vi "Test Case Runner.vi"(0 "Problem":T1, 1 "Numeric 2":dbl, 2 "Numeric Array 2":dbl[](array[numeric]), 3 "String 2":string, 4 "String Array 2":string[](array[string]), 5 "Iterator":i32, 8 "TestCases Folder":path, 9 "Send Input?":bool) -> (15 "Numeric":dbl, 16 "Numeric Array":dbl[](array[numeric]), 17 "String":string, 18 "String Array":string[](array[string]), 19 "Accepted":bool)   [LabVIEW 2014]
uses:
  Main Contest/Problem.ctl
  <vilib>/Utility/file.llb/Read From Spreadsheet File (string).vi
  <vilib>/Utility/file.llb/Read From Spreadsheet File (DBL).vi
panel:
  out "E":path=path "C:/Users/Justin/Desktop/LabVIEW-Rank/Offline Judge/TestCases/Test A.csv"
  out "D":path=path "C:/Users/Justin/Desktop/LabVIEW-Rank/Offline Judge/TestCases/Test A.csv"
  out "C":path=path "C:/Users/Justin/Desktop/LabVIEW-Rank/Offline Judge/TestCases/Test A.csv"
  out "B":path=path "C:/Users/Justin/Desktop/LabVIEW-Rank/Offline Judge/TestCases/Test A.csv"
  out "A":path=path "C:/Users/Justin/Desktop/LabVIEW-Rank/Offline Judge/TestCases/Test A.csv"
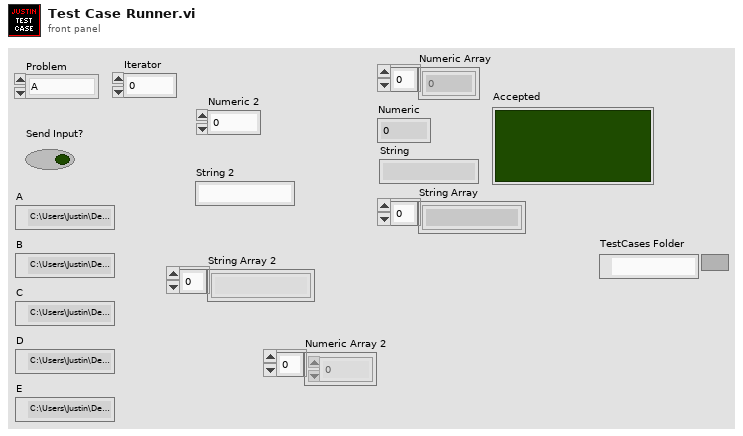
[diagram p1: front panel]
types:
  T1 = typedef "Problem.ctl" = enum16{"A", "B", "C", "D", "E"}
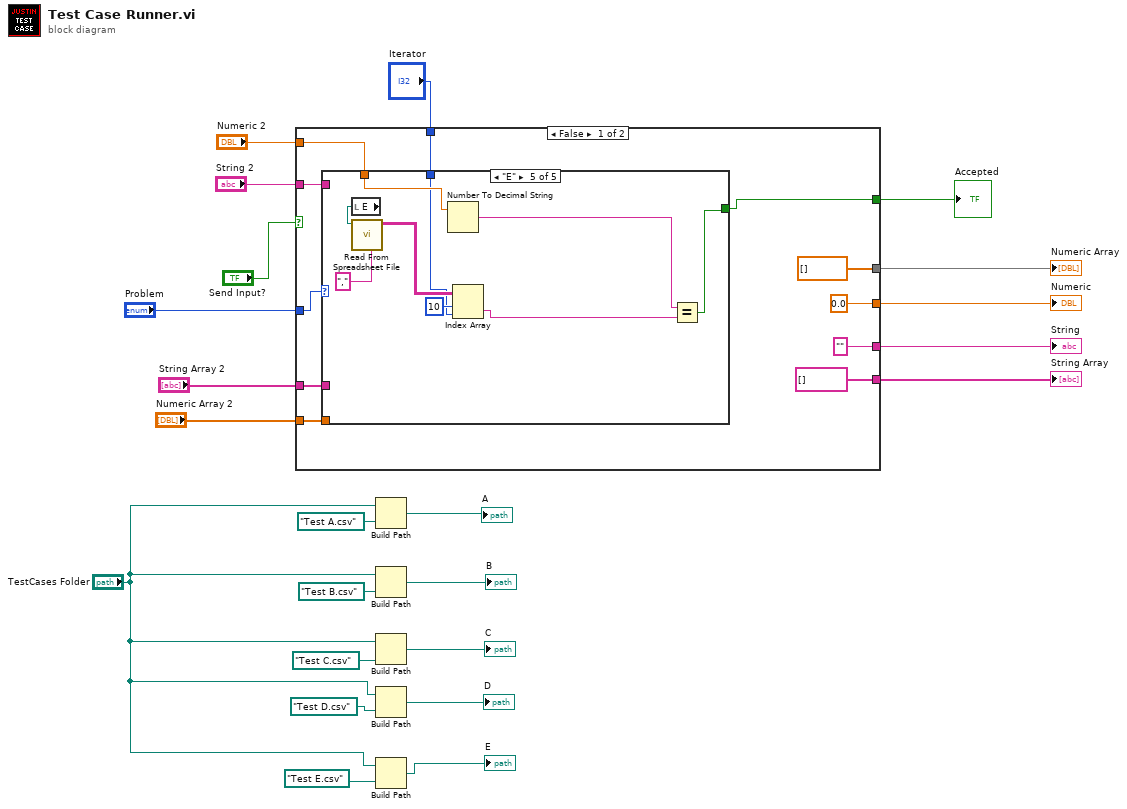
[diagram p0: block diagram]
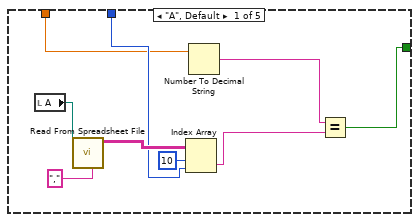
[diagram p2: hidden frame]
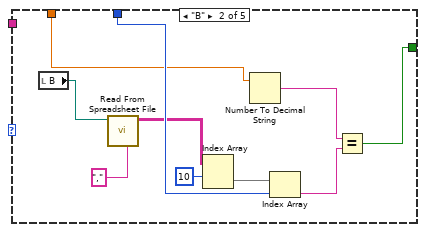
[diagram p3: hidden frame]
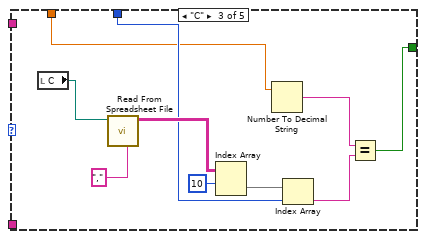
[diagram p4: hidden frame]
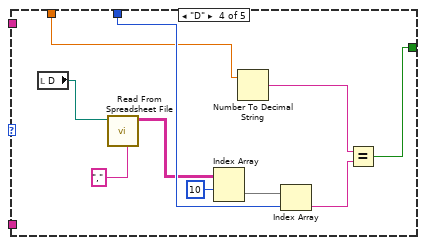
[diagram p5: hidden frame]
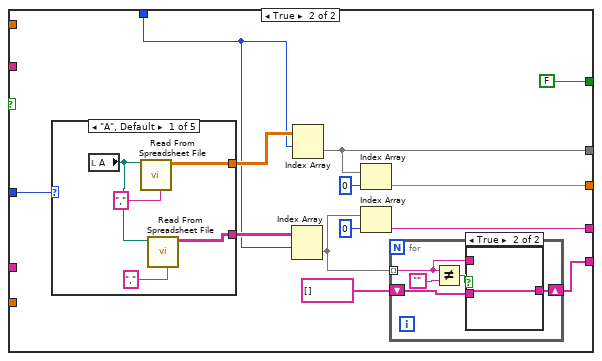
[diagram p6: hidden frame]
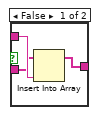
[diagram p7: hidden frame]
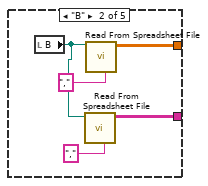
[diagram p8: hidden frame]
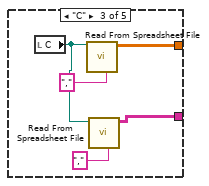
[diagram p9: hidden frame]
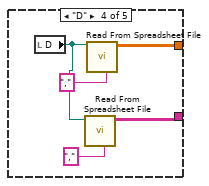
[diagram p10: hidden frame]
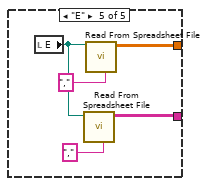
[diagram p11: hidden frame]
diagram:
  n1 = case shown="False" "Send Input?" {
    tunnel: "Problem" -> [w34 w95]
    tunnel: [w24 FALSE] -> w21
    tunnel: "Iterator" -> [w25 w88]
    tunnel: [dbl[] [] ("all rows") w92] -> w19
    tunnel: [0.0 w90] -> w18
    tunnel: [string[] [] ("all rows") w83] -> w16
    tunnel: ["" ("String") w86] -> w17
    tunnel: "Numeric 2" -> [w29 _]
    tunnel: "String Array 2" -> [w28 _]
    tunnel: "Numeric Array 2" -> [w27 _]
    tunnel: "String 2" -> [w26 _]
    frame False {
      n2 = case shown="\"E\"" w34 {
        tunnel: w29 -> [w36 w46 w56 w64 w79]
        tunnel: w28 -> [_ _ _ _ _]
        tunnel: w27 -> [_ _ _ _ _]
        tunnel: w26 -> [_ _ _ _ _]
        tunnel: w25 -> [w39 w49 w58 w69 w75]
        tunnel: [w40 w47 w57 w67 w81] -> w24
        frame "A", Default {
          n3 = local read "A"() -> (w43:path)
          n4 = call-poly <vilib>:"Read From Spreadsheet File.vi"("delimiter (\\t)"="," ("delimiter (\\t)"), "file path (dialog if empty)"=w43) -> ("all rows"=w42:string[][])  [unwired: 5 in, 4 out]
          n5 = Index Array(array=w42, index (row)=10, index (col)=w39) -> (element=w38:string)
          n6 = Number To Decimal String(number=w36) -> (decimal integer string=w35:string)  [unwired: 1 in]
          n7 = Equal?(x=w35, y=w38) -> (x = y?=w40:bool)
        }
        frame "B" {
          n8 = local read "B"() -> (w53:path)
          n9 = call-poly <vilib>:"Read From Spreadsheet File.vi"("delimiter (\\t)"="," ("delimiter (\\t)"), "file path (dialog if empty)"=w53) -> ("all rows"=w48:string[][])  [unwired: 5 in, 4 out]
          n10 = Index Array(array=w48, index (row)=10) -> (element=w51:string[])  [unwired: 1 in]
          n11 = Number To Decimal String(number=w46) -> (decimal integer string=w45:string)  [unwired: 1 in]
          n12 = Index Array(array=w51, index=w49) -> (element=w52:string)
          n13 = Equal?(x=w45, y=w52) -> (x = y?=w47:bool)
        }
        frame "C" {
          n14 = local read "C"() -> (w63:path)
          n15 = call-poly <vilib>:"Read From Spreadsheet File.vi"("delimiter (\\t)"="," ("delimiter (\\t)"), "file path (dialog if empty)"=w63) -> ("all rows"=w59:string[][])  [unwired: 5 in, 4 out]
          n16 = Index Array(array=w59, index (row)=10) -> (element=w61:string[])  [unwired: 1 in]
          n17 = Number To Decimal String(number=w56) -> (decimal integer string=w55:string)  [unwired: 1 in]
          n18 = Index Array(array=w61, index=w58) -> (element=w62:string)
          n19 = Equal?(x=w55, y=w62) -> (x = y?=w57:bool)
        }
        frame "D" {
          n20 = local read "D"() -> (w73:path)
          n21 = call-poly <vilib>:"Read From Spreadsheet File.vi"("delimiter (\\t)"="," ("delimiter (\\t)"), "file path (dialog if empty)"=w73) -> ("all rows"=w68:string[][])  [unwired: 5 in, 4 out]
          n22 = Index Array(array=w68, index (row)=10) -> (element=w71:string[])  [unwired: 1 in]
          n23 = Number To Decimal String(number=w64) -> (decimal integer string=w65:string)  [unwired: 1 in]
          n24 = Index Array(array=w71, index=w69) -> (element=w70:string)
          n25 = Equal?(x=w65, y=w70) -> (x = y?=w67:bool)
        }
        frame "E" {
          n26 = local read "E"() -> (w82:path)
          n27 = call-poly <vilib>:"Read From Spreadsheet File.vi"("delimiter (\\t)"="," ("delimiter (\\t)"), "file path (dialog if empty)"=w82) -> ("all rows"=w77:string[][])  [unwired: 5 in, 4 out]
          n28 = Number To Decimal String(number=w79) -> (decimal integer string=w78:string)  [unwired: 1 in]
          n29 = Index Array(array=w77, index (row)=10, index (col)=w75) -> (element=w74:string)
          n30 = Equal?(x=w78, y=w74) -> (x = y?=w81:bool)
        }
      }
    }
    frame True {
      n31 = case shown="\"A\", Default" w95 {
        tunnel: [w108 w114 w117 w123 w127] -> w93
        tunnel: [w107 w112 w118 w124 w128] -> w89
        frame "A", Default {
          n32 = local read "A"() -> (w109:path)
          n33 = call-poly <vilib>:"Read From Spreadsheet File.vi"("delimiter (\\t)"="," ("delimiter (\\t)"), "file path (dialog if empty)"=w109) -> ("all rows"=w108:dbl[][])  [unwired: 5 in, 4 out]
          n34 = call-poly <vilib>:"Read From Spreadsheet File.vi"("delimiter (\\t)"="," ("delimiter (\\t)"), "file path (dialog if empty)"=w109) -> ("all rows"=w107:string[][])  [unwired: 5 in, 4 out]
        }
        frame "B" {
          n35 = local read "B"() -> (w113:path)
          n36 = call-poly <vilib>:"Read From Spreadsheet File.vi"("delimiter (\\t)"="," ("delimiter (\\t)"), "file path (dialog if empty)"=w113) -> ("all rows"=w112:string[][])  [unwired: 5 in, 4 out]
          n37 = call-poly <vilib>:"Read From Spreadsheet File.vi"("delimiter (\\t)"="," ("delimiter (\\t)"), "file path (dialog if empty)"=w113) -> ("all rows"=w114:dbl[][])  [unwired: 5 in, 4 out]
        }
        frame "C" {
          n38 = local read "C"() -> (w119:path)
          n39 = call-poly <vilib>:"Read From Spreadsheet File.vi"("delimiter (\\t)"="," ("delimiter (\\t)"), "file path (dialog if empty)"=w119) -> ("all rows"=w117:dbl[][])  [unwired: 5 in, 4 out]
          n40 = call-poly <vilib>:"Read From Spreadsheet File.vi"("delimiter (\\t)"="," ("delimiter (\\t)"), "file path (dialog if empty)"=w119) -> ("all rows"=w118:string[][])  [unwired: 5 in, 4 out]
        }
        frame "D" {
          n41 = local read "D"() -> (w122:path)
          n42 = call-poly <vilib>:"Read From Spreadsheet File.vi"("delimiter (\\t)"="," ("delimiter (\\t)"), "file path (dialog if empty)"=w122) -> ("all rows"=w124:string[][])  [unwired: 5 in, 4 out]
          n43 = call-poly <vilib>:"Read From Spreadsheet File.vi"("delimiter (\\t)"="," ("delimiter (\\t)"), "file path (dialog if empty)"=w122) -> ("all rows"=w123:dbl[][])  [unwired: 5 in, 4 out]
        }
        frame "E" {
          n44 = local read "E"() -> (w129:path)
          n45 = call-poly <vilib>:"Read From Spreadsheet File.vi"("delimiter (\\t)"="," ("delimiter (\\t)"), "file path (dialog if empty)"=w129) -> ("all rows"=w128:string[][])  [unwired: 5 in, 4 out]
          n46 = call-poly <vilib>:"Read From Spreadsheet File.vi"("delimiter (\\t)"="," ("delimiter (\\t)"), "file path (dialog if empty)"=w129) -> ("all rows"=w127:dbl[][])  [unwired: 5 in, 4 out]
        }
      }
      n47 = Index Array(array=w89, index (row)=w88) -> (element=w85:string[])  [unwired: 1 in]
      n48 = Index Array(array=w93, index (row)=w88) -> (element=w92:dbl[])  [unwired: 1 in]
      n49 = Index Array(array=w92, index=0) -> (element=w90:dbl)
      n50 = Index Array(array=w85, index=0) -> (element=w86:string)
      n51 = for {
        tunnel: w85 -> [w98] mode=indexing
        shift-right: [w96] -> w83
        shift-left: string[] [] ("subarray") -> [w97]
        n52 = Not Equal?(x=w98, y="") -> (x != y?=w99:bool)
        n53 = case shown="True" w99 {
          tunnel: w98 -> [w103 _]
          tunnel: w97 -> [w102 w104]
          tunnel: [w101 w104] -> w96
          frame False {
            n54 = Insert Into Array(array=w102, new element=w103) -> (w101:string[])  [unwired: 1 in]
          }
          frame True {
          }
        }
      }
    }
  }
  "Accepted" <- w21
  "Numeric Array" <- w19
  "Numeric" <- w18
  "String" <- w17
  "String Array" <- w16
  n55 = Build Path(base path="TestCases Folder", name or relative path=path "Test A.csv" ("file path (dialog if empty)")) -> (appended path=→"A":path)
  n56 = Build Path(base path="TestCases Folder", name or relative path=path "Test B.csv" ("file path (dialog if empty)")) -> (appended path=→"B":path)
  n57 = Build Path(base path="TestCases Folder", name or relative path=path "Test C.csv" ("file path (dialog if empty)")) -> (appended path=→"C":path)
  n58 = Build Path(base path="TestCases Folder", name or relative path=path "Test D.csv" ("file path (dialog if empty)")) -> (appended path=→"D":path)
  n59 = Build Path(base path="TestCases Folder", name or relative path=path "Test E.csv" ("file path (dialog if empty)")) -> (appended path=→"E":path)
